vi "Config-Delete Section.vi"(0 "configuration file path":path, 2 "section":string, 11 "error in (no error)":errorcluster) -> (4 "file path":path, 15 "error out":errorcluster)   [LabVIEW 2020]
uses:
  <vilib>/Utility/config.llb/NI_LVConfig.lvlib
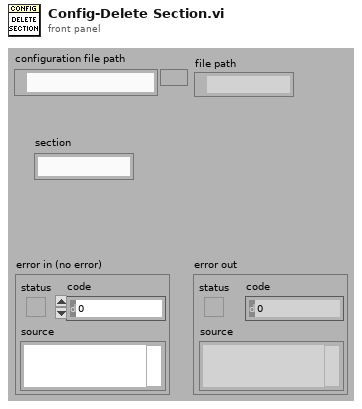
[diagram p1: front panel]
types:
  T1 = typedef "NI_LVConfig.lvlib/Config Data RefNum.ctl" = refnum<k1>
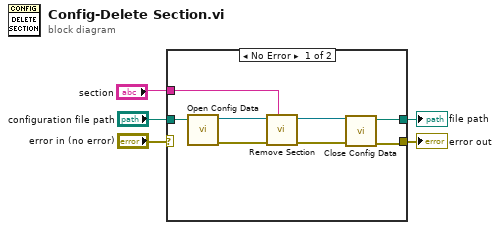
[diagram p0: block diagram]
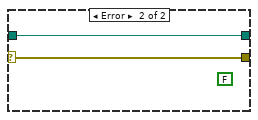
[diagram p2: hidden frame]
diagram:
  n1 = case shown="No Error" "error in (no error)" {
    selector: "error in (no error)" -> [_ w15]
    tunnel: [w13 w15] -> w5
    tunnel: "configuration file path" -> [w12 w14]
    tunnel: [w11 w14] -> w2
    tunnel: "section" -> [w7 _]
    frame No Error {
      n2 = call <vilib>:"Open Config Data.vi"("configuration file path"=w12) -> ("error out"=w8:errorcluster, "refnum"=w10:T1)  [unwired: 8 in, 1 out]
      n3 = call <vilib>:"Remove Section.vi"("section"=w7, "error in (no error)"=w8, "refnum"=w10) -> ("error out"=w6:errorcluster, "refnum out"=w9:T1)  [unwired: 6 in, 1 out]
      n4 = call <vilib>:"Close Config Data.vi"("error in (no error)"=w6, "refnum"=w9) -> ("error out"=w13:errorcluster, "file path"=w11:path)  [unwired: 8 in]
    }
    frame Error {
      (unwired) FALSE ("found?")
    }
  }
  "error out" <- w5
  "file path" <- w2
